vi "ABOR.vi"(8 "error in (no error)":errorcluster, 11 "FTP in":refnum<class "FTP.lvclass">) -> (0 "error out":errorcluster, 3 "FTP out":refnum<class "FTP.lvclass">)   [LabVIEW 2013, in "FTP.lvlib" / "FTP.lvclass"]
uses:
  FTP.lvclass
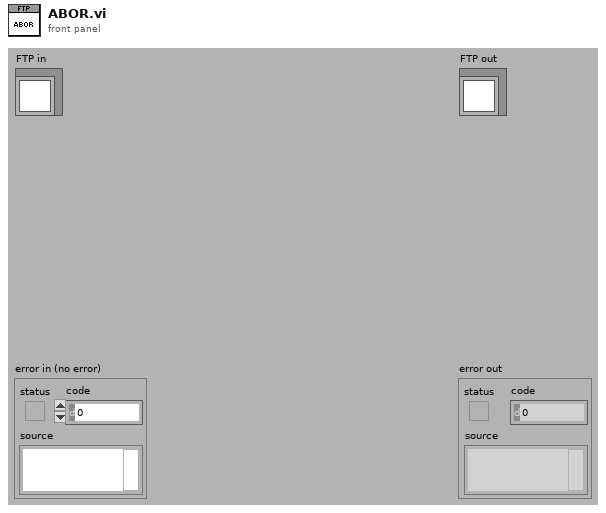
[diagram p1: front panel]
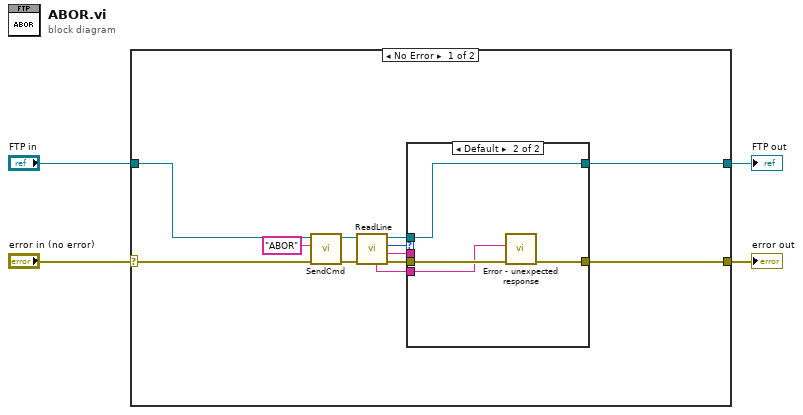
[diagram p0: block diagram]
diagram:
  n1 = case shown="No Error" "error in (no error)" {
    selector: "error in (no error)" -> [w9 w24]
    tunnel: [w7 w24] -> w3
    tunnel: [w8 w23] -> w1
    tunnel: "FTP in" -> [w10 w23]
    frame No Error {
      n2 = call "SendCmd.vi"("error in (no error)"=w9, "cmd"="ABOR", "FTP in"=w10) -> ("error out"=w16:errorcluster, "FTP out"=w15:refnum<class "FTP.lvclass">)  [unwired: 7 in]
      n3 = call "ReadLine.vi"("error in (no error)"=w16, "FTP in"=w15) -> ("error out"=w12:errorcluster, "Line"=w11:string, "code"=w13:i32, "FTP out"=w14:refnum<class "FTP.lvclass">, "Full Line"=w5:string)  [unwired: 5 in]
      n4 = case shown="Default" w13 {
        tunnel: w14 -> [w18 w22]
        tunnel: w12 -> [w17 w21]
        tunnel: [w17 w20] -> w7
        tunnel: [w18 w22] -> w8
        tunnel: w11 -> [_ _]
        tunnel: w5 -> [_ w19]
        frame 250 {
        }
        frame Default {
          n5 = call "Error - unexpected response.vi"("error in (no error)"=w21, "Full Response"=w19) -> ("error out"=w20:errorcluster)  [unwired: 9 in]
        }
      }
    }
    frame Error {
    }
  }
  "error out" <- w3
  "FTP out" <- w1
